vi "Adapt to inputs.vi"(3 "Term Types":T1[](array[typedef]), 4 "XRef":refnum<vi>, 5 "State In":T4) -> (0 "Reply":string[](array[string]), 2 "State Out":T4)   [LabVIEW 2012, in "OpenG FilterArray.xnode"]
uses:
  OpenG FilterArray.xnode
  State.ctl
  <vilib>/XNodeSupport/XNodeTermTypeIDPair.ctl
  <vilib>/XNodeSupport/XNodeType.ctl
  <vilib>/XNodeSupport/XNodeString.ctl
  <vilib>/Utility/VariantDataType/Type.ctl
  <vilib>/Utility/VariantDataType/VariantType.lvlib
  <vilib>/XNodeSupport/NI_XNodeSupport.lvlib
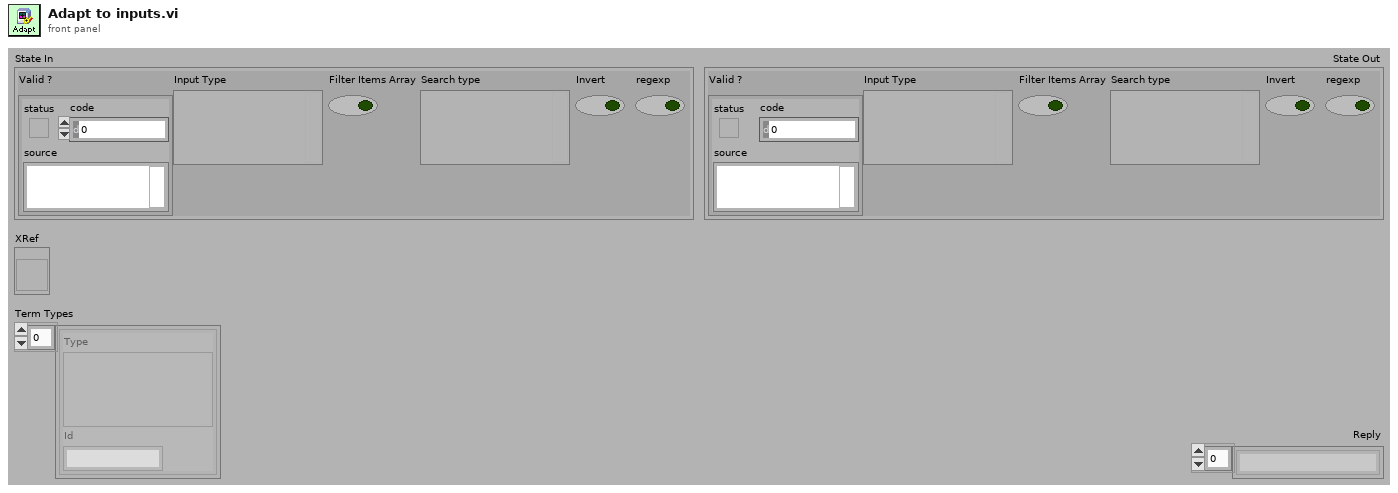
[diagram p1: front panel]
types:
  T1 = typedef "NI_XNodeSupport.lvlib/XNodeTermTypeIDPair.ctl" = cluster{"Type":T2, "Id":T3}
  T2 = typedef "NI_XNodeSupport.lvlib/XNodeType.ctl" = variant
  T3 = typedef "NI_XNodeSupport.lvlib/XNodeString.ctl" = string
  T4 = typedef "OpenG FilterArray.xnode/State.ctl" = cluster{"Valid ?":errorcluster, "Input Type":variant, "Filter Items Array":bool, "Search type":variant, "Invert":bool, "regexp":bool}
  T5 = typedef "VariantType.lvlib/Type.ctl" = enum8{"Invalid Type", "Void", "I8", "I16", "I32", "I64", "U8", "U16", "U32", "U64", "Single Float", "Double Float", "Extended Float", "Single Complex", "Double Complex", "Extended Complex", "Enum U8", "Enum U16", "Enum U32", "Enum U64", "Single Float With Unit", "Double Float With Unit", "Extended Float With Unit", "Single Complex with Unit", "Double Complex with Unit", "Extended Complex with Unit", "Boolean", "String", "Path", "Picture", "Tag", "Array", "Cluster", "Variant", "LV Variant", "Waveform", "Timestamp", "Digital Waveform", "Digital Data", "ExpressData", "Refnum", "External Data", "VI", "Poly VI", "LabVIEW Class Instance", "Fixed Point"}
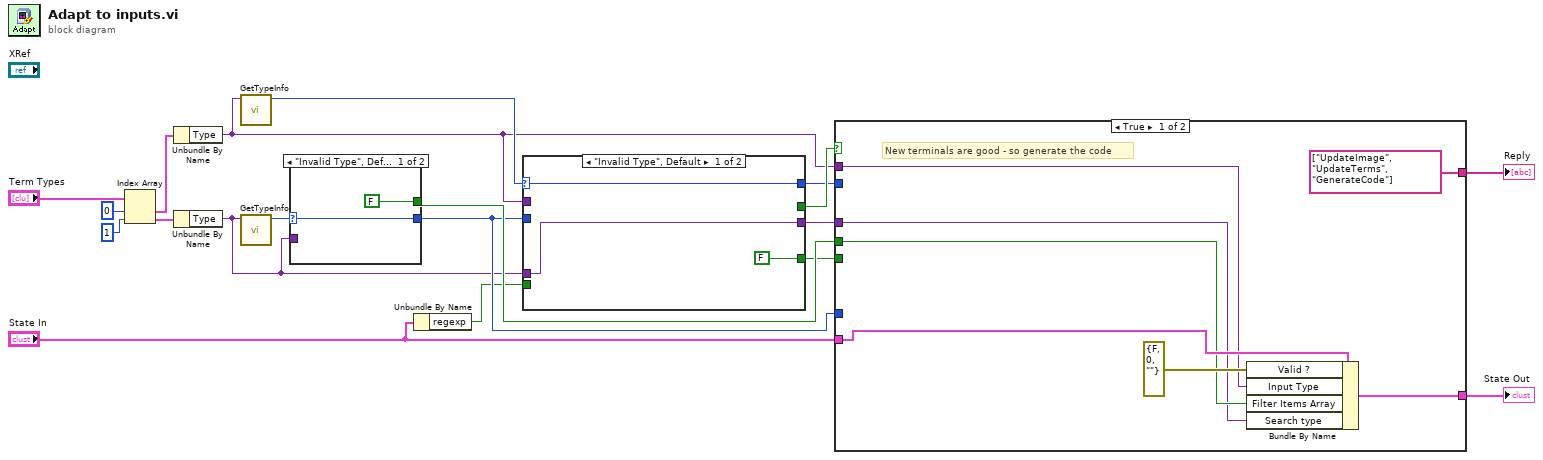
[diagram p0: block diagram]
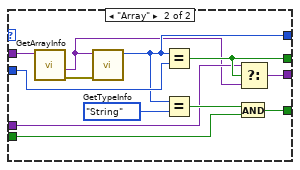
[diagram p2: hidden frame]
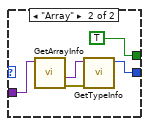
[diagram p3: hidden frame]
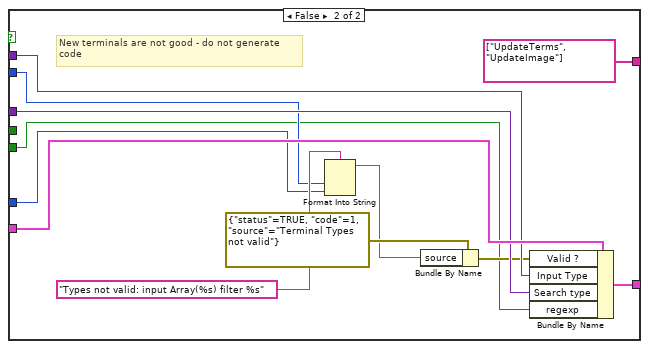
[diagram p4: hidden frame]
diagram:
  n1 = Index Array(array="Term Types", index #1=0 ("Dimension"), index #2=1 ("index")) -> (element #1=w15:T1, element #2=w13:T1)
  n2 = Unbundle By Name(w15) -> ("Type"=w6:T2)
  n3 = Unbundle By Name(w13) -> ("Type"=w2:T2)
  n4 = call <vilib>:"GetTypeInfo.vi"("Variant"=w6) -> ("Type Enum"=w11:T5)  [unwired: 1 in, 9 out]
  n5 = call <vilib>:"GetTypeInfo.vi"("Variant"=w2) -> ("Type Enum"=w12:T5)  [unwired: 1 in, 9 out]
  n6 = case shown="\"Invalid Type\", Default" w12 {
    selector: w12 -> [w21 _]
    tunnel: w2 -> [_ w26]
    tunnel: [w21 w23] -> w8
    tunnel: [FALSE TRUE] -> w9
    frame "Invalid Type", Default {
    }
    frame "Array" {
      n7 = call <vilib>:"GetArrayInfo.vi"("Variant"=w26) -> ("error out"=w25:errorcluster, "ArrayElement"=w24:variant)  [unwired: 1 in, 8 out]
      n8 = call <vilib>:"GetTypeInfo.vi"("error in (no error)"=w25, "Variant"=w24) -> ("Type Enum"=w23:T5)  [unwired: 9 out]
    }
  }
  n9 = Unbundle By Name("State In") -> ("regexp"=w4:bool)
  n10 = case shown="\"Invalid Type\", Default" w11 {
    selector: w11 -> [w29 _]
    tunnel: w6 -> [_ w41]
    tunnel: [_ w33] -> w10
    tunnel: w8 -> [_ w39]
    tunnel: [w29 w38] -> w7
    tunnel: [FALSE w35] -> w3
    tunnel: w4 -> [_ w36]
    tunnel: w2 -> [w27 w32]
    tunnel: [w27 w30] -> w1
    frame "Invalid Type", Default {
    }
    frame "Array" {
      n11 = call <vilib>:"GetArrayInfo.vi"("Variant"=w41) -> ("error out"=w40:errorcluster, "ArrayElement"=w31:variant)  [unwired: 1 in, 8 out]
      n12 = call <vilib>:"GetTypeInfo.vi"("error in (no error)"=w40, "Variant"=w31) -> ("Type Enum"=w38:T5)  [unwired: 9 out]
      n13 = Equal?(x=w38, y=w39) -> (x = y?=w33:bool)
      n14 = Equal?(x=w38, y=Type."String") -> (x = y?=w34:bool)
      n15 = And(x=w34, y=w36) -> (x .and. y?=w35:bool)
      n16 = Select(t=w32, s=w33, f=w31) -> (s? t:f=w30:T2)
    }
  }
  n17 = case shown="True" w10 {
    tunnel: "State In" -> [w48 w60]
    tunnel: [w46 w58] -> w19
    tunnel: [string[] ["UpdateImage", "UpdateTerms", "GenerateCode"] ("Reply") string[] ["UpdateTerms", "UpdateImage"] ("Reply")] -> w18
    tunnel: w6 -> [w44 w56]
    tunnel: w9 -> [w43 _]
    tunnel: w1 -> [w42 w55]
    tunnel: w8 -> [_ w51]
    tunnel: w7 -> [_ w50]
    tunnel: w3 -> [_ w49]
    frame True {
      # "New terminals are good - so generate the code"
      n18 = Bundle By Name(cluster=w48, "Valid ?"=errorcluster {"status"=FALSE, "code"=0, "source"=""}, "Input Type"=w44, "Filter Items Array"=w43, "Search type"=w42) -> (w46:T4)
    }
    frame False {
      # "New terminals are not good - do not generate\ncode"
      n19 = Format Into String(format string="Types not valid: input Array(%s) filter %s", w50, w51) -> (resulting string=w52:string)  [unwired: 2 in, 1 out]
      n20 = Bundle By Name(cluster=errorcluster {"status"=TRUE, "code"=1, "source"="Terminal Types not valid"} ("Valid ?"), "source"=w52) -> (w54:errorcluster)
      n21 = Bundle By Name(cluster=w60, "Valid ?"=w54, "Input Type"=w56, "Search type"=w55, "regexp"=w49) -> (w58:T4)
    }
  }
  "Reply" <- w18
  "State Out" <- w19
